vi "CODMn 随机数出数.vi"(4 "公式":cluster{"X^2":dbl, "X":dbl, "B":dbl}, 5 "测试模式":enum16{"水样测试", "零点核查", "跨度核查"}(ring), 8 "信号值原始值":dbl, 9 "原始值":dbl) -> (1 "随机数？":bool, 2 "信号值":u16, 3 "取值输出":dbl)   [LabVIEW 2016]
uses:
  Holding Var.vi
  Process var.vi
  random number/random number.lvlib
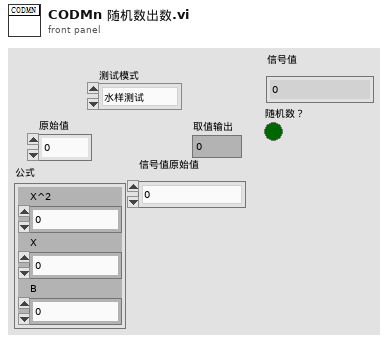
[diagram p1: front panel]
types:
  T1 = cluster{"水样参数输出":cluster{"mean":dbl, "变异系数":dbl, "随机数？":bool}, "零点参数输出":cluster{"mean":dbl, "变异系数":dbl, "随机数？":bool}, "跨度参数输出":cluster{"mean":dbl, "变异系数":dbl, "随机数？":bool}}
  T2 = cluster{"水样测试":cluster{"参数输入":cluster{"采样模式":enum16{"自动采样", "手动采样"}, "采样点数":i32, "变异系数设定值":dbl, "重新取值百分比":dbl, "偏差模式":enum16{"相对偏差", "绝对偏差"}, "相对偏差百分比":dbl, "绝对偏差值":dbl}, "采样值":dbl[], "启用":bool}, "零点核查":cluster{"参数输入":cluster{"采样模式":enum16{"自动采样", "手动采样"}, "采样点数":i32, "变异系数设定值":dbl, "重新取值百分比":dbl, "偏差模式":enum16{"相对偏差", "绝对偏差"}, "相对偏差百分比":dbl, "绝对偏差值":dbl}, "采样值":dbl[], "启用":bool}, "跨度核查":cluster{"参数输入":cluster{"采样模式":enum16{"自动采样", "手动采样"}, "采样点数":i32, "变异系数设定值":dbl, "重新取值百分比":dbl, "偏差模式":enum16{"相对偏差", "绝对偏差"}, "相对偏差百分比":dbl, "绝对偏差值":dbl}, "采样值":dbl[], "启用":bool}}
  T3 = cluster{"采样模式":enum16{"自动采样", "手动采样"}, "采样点数":i32, "变异系数设定值":dbl, "重新取值百分比":dbl, "偏差模式":enum16{"相对偏差", "绝对偏差"}, "相对偏差百分比":dbl, "绝对偏差值":dbl}
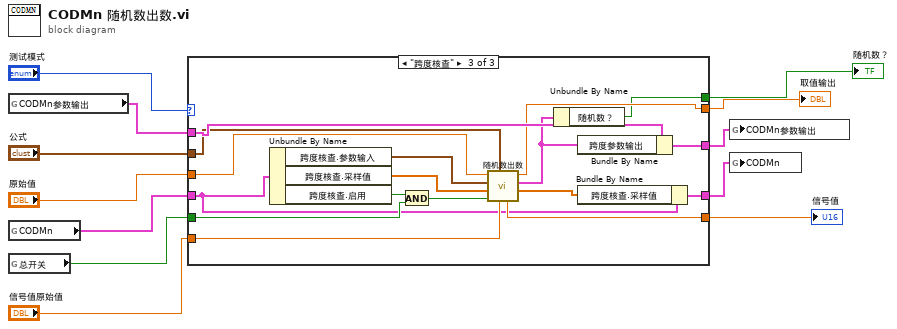
[diagram p0: block diagram]
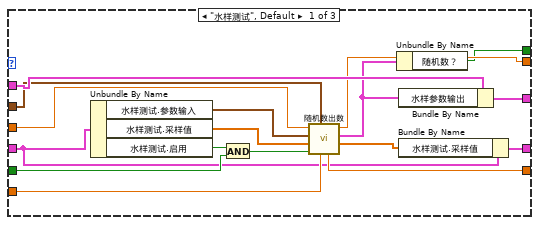
[diagram p2: hidden frame]
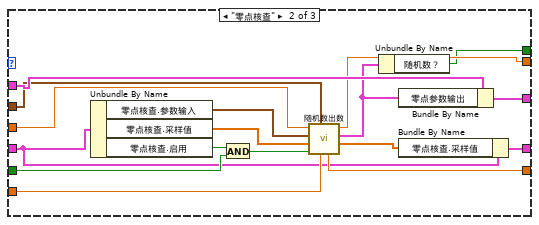
[diagram p3: hidden frame]
diagram:
  n1 = global read "Process var.vi" "CODMn参数输出"() -> (w11:T1)
  n2 = global read "Holding Var.vi" "CODMn"() -> (w12:T2)
  n3 = global read "Holding Var.vi" "总开关"() -> (w6:bool)
  n4 = case shown="\"跨度核查\"" "测试模式" {
    tunnel: w12 -> [w17 w34 w51]
    tunnel: w11 -> [w27 w44 w61]
    tunnel: [w26 w43 w60] -> w10
    tunnel: "原始值" -> [w25 w42 w59]
    tunnel: [w24 w41 w58] -> w7
    tunnel: w6 -> [w23 w40 w57]
    tunnel: "公式" -> [w20 w37 w54]
    tunnel: "信号值原始值" -> [w19 w36 w53]
    tunnel: [w18 w35 w52] -> w3
    tunnel: [w16 w33 w50] -> w2
    tunnel: [w13 w30 w47] -> w1
    frame "水样测试", Default {
      n5 = Unbundle By Name(w17) -> ("水样测试.参数输入"=w29:T3, "水样测试.采样值"=w28:dbl[], "水样测试.启用"=w22:bool)
      n6 = And(x=w22, y=w23) -> (x .and. y?=w21:bool)
      n7 = call "随机数出数.vi"("信号值原始值"=w19, "公式"=w20, "启用"=w21, "采样值"=w28, "参数输入"=w29, "监测值原始值"=w25) -> ("采样值输出"=w15:dbl[], "参数输出"=w14:cluster{"mean":dbl, "变异系数":dbl, "随机数？":bool}, "取值输出"=w24:dbl, "信号值"=w18:dbl)  [unwired: 2 in]
      n8 = Unbundle By Name(w14) -> ("随机数？"=w13:bool)
      n9 = Bundle By Name(cluster=w27, "水样参数输出"=w14) -> (w26:T1)
      n10 = Bundle By Name(cluster=w17, "水样测试.采样值"=w15) -> (w16:T2)
    }
    frame "零点核查" {
      n11 = Unbundle By Name(w34) -> ("零点核查.参数输入"=w46:T3, "零点核查.采样值"=w45:dbl[], "零点核查.启用"=w39:bool)
      n12 = And(x=w39, y=w40) -> (x .and. y?=w38:bool)
      n13 = call "随机数出数.vi"("信号值原始值"=w36, "公式"=w37, "启用"=w38, "采样值"=w45, "参数输入"=w46, "监测值原始值"=w42) -> ("采样值输出"=w32:dbl[], "参数输出"=w31:cluster{"mean":dbl, "变异系数":dbl, "随机数？":bool}, "取值输出"=w41:dbl, "信号值"=w35:dbl)  [unwired: 2 in]
      n14 = Unbundle By Name(w31) -> ("随机数？"=w30:bool)
      n15 = Bundle By Name(cluster=w44, "零点参数输出"=w31) -> (w43:T1)
      n16 = Bundle By Name(cluster=w34, "零点核查.采样值"=w32) -> (w33:T2)
    }
    frame "跨度核查" {
      n17 = Unbundle By Name(w51) -> ("跨度核查.参数输入"=w63:T3, "跨度核查.采样值"=w62:dbl[], "跨度核查.启用"=w56:bool)
      n18 = And(x=w56, y=w57) -> (x .and. y?=w55:bool)
      n19 = call "随机数出数.vi"("信号值原始值"=w53, "公式"=w54, "启用"=w55, "采样值"=w62, "参数输入"=w63, "监测值原始值"=w59) -> ("采样值输出"=w49:dbl[], "参数输出"=w48:cluster{"mean":dbl, "变异系数":dbl, "随机数？":bool}, "取值输出"=w58:dbl, "信号值"=w52:dbl)  [unwired: 2 in]
      n20 = Unbundle By Name(w48) -> ("随机数？"=w47:bool)
      n21 = Bundle By Name(cluster=w61, "跨度参数输出"=w48) -> (w60:T1)
      n22 = Bundle By Name(cluster=w51, "跨度核查.采样值"=w49) -> (w50:T2)
    }
  }
  "取值输出" <- w7
  "信号值" <- w3
  "随机数？" <- w1
  n23 = global write "Process var.vi" "CODMn参数输出"(w10) -> ()
  n24 = global write "Holding Var.vi" "CODMn"(w2) -> ()
